vi "SaveTree.vi"(8 "error in":errorcluster, 11 "TreeControl in":refnum<vi>) -> (0 "error out":errorcluster)   [LabVIEW 2014]
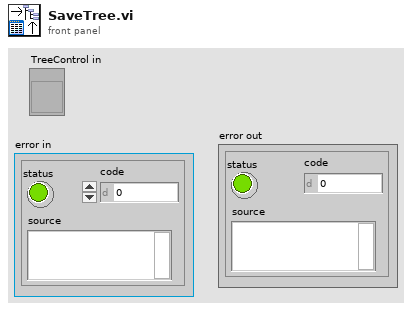
[diagram p1: front panel]
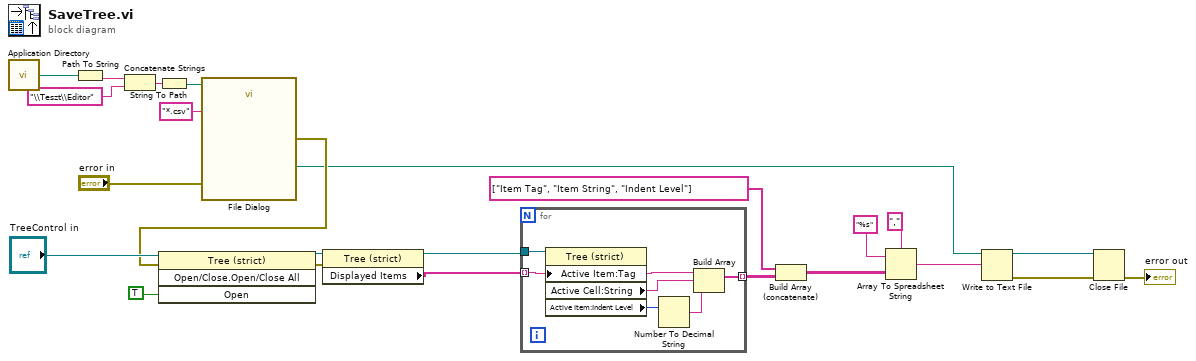
[diagram p0: block diagram]
diagram:
  n1 = call <vilib>:"Application Directory.vi"() -> ("Application Directory"=w14:path)
  n2 = Path To String(path=w14) -> (string=w17:string)
  n3 = Concatenate Strings(w17, "\\Teszt\\Editor" ("prompt (Choose or enter file path)")) -> (w16:string)
  n4 = String To Path(string=w16) -> (path=w13:path)
  n5 = call "File Dialog"("start path"=w13, "error in"="error in", "pattern (all files)"="*.csv") -> ("selected path"=w10:path, "error out"=w12:errorcluster)  [unwired: 9 in, 2 out]
  n6 = invoke class="Tree (strict)" method="Open/Close.Open/Close All"(reference="TreeControl in", error in=w12, "Open"=TRUE) -> (reference out=w23:refnum<vi>, error out=w11:errorcluster)  [unwired: 1 in, 2 out]
  n7 = property class="Tree (strict)"(reference=w23, error in=w11) -> (reference out=w7:refnum<vi>, "Displayed Items"=w6:string[])  [unwired: 1 out]
  n8 = for {
    tunnel: w6 -> [w29] mode=indexing
    tunnel: w7 -> [w30]
    tunnel: [w28] -> w9 mode=indexing
    n9 = property class="Tree (strict)"(reference=w30, "Active Item:Tag"=w29) -> ("Active Cell:String"=w26:string, "Active Item:Indent Level"=w27:i32)  [unwired: 1 in, 2 out]
    n10 = Number To Decimal String(number=w27) -> (decimal integer string=w25:string)  [unwired: 1 in]
    n11 = Build Array(w29, w26, w25) -> (w28:string[])
  }
  n12 = Build Array (concatenate)(string[] ["Item Tag", "Item String", "Indent Level"], w9) -> (w5:string[][])
  n13 = Array To Spreadsheet String(delimiter (Tab)=",", array=w5, 3:"%s" ("format string")) -> (spreadsheet string=w21:string)
  n14 = Write to Text File(file (use dialog)=w10, text=w21) -> (refnum out=w3:refnum<file>, error out=w4:errorcluster)  [unwired: 2 in, 1 out]
  n15 = Close File(refnum=w3, error in=w4) -> (error out=→"error out":errorcluster)  [unwired: 1 out]
